vi "Answer Eval.vi"(5 "Answer Format":enum16{"Wfm", "Sim Param"}(ring), 6 "Error Deviation (%)":dbl=5.0 format="%#_13g", 7 "Exercise Number":T1, 8 "error in":errorcluster, 9 "Data In":variant, 11 "Exercise Folder Path":path) -> (0 "error out":errorcluster, 2 "Response Array":bool[](array[boolean]), 3 "path":path)   [LabVIEW 2014]
uses:
  Ctls/ExerciseNumeration.ctl
  Ctls/t1q1.ctl
  Ctls/RCSim Controls.ctl
  Ctls/t1q2.ctl
  <vilib>/express/express analysis/Spectral/Block/exnSpectralBlock spectral measurements peak poly.vi
  <vilib>/express/express analysis/Spectral/Block/exnSpectralBlock spectral measurements peak WFM.vi
  <vilib>/express/express analysis/Spectral/XNode/ExpressSpectralMeasurementsBlockNode.xnode
panel:
  out "Waveform In FFT":cluster{"f0":dbl, "df":dbl, "magnitude":dbl[]}(graph)
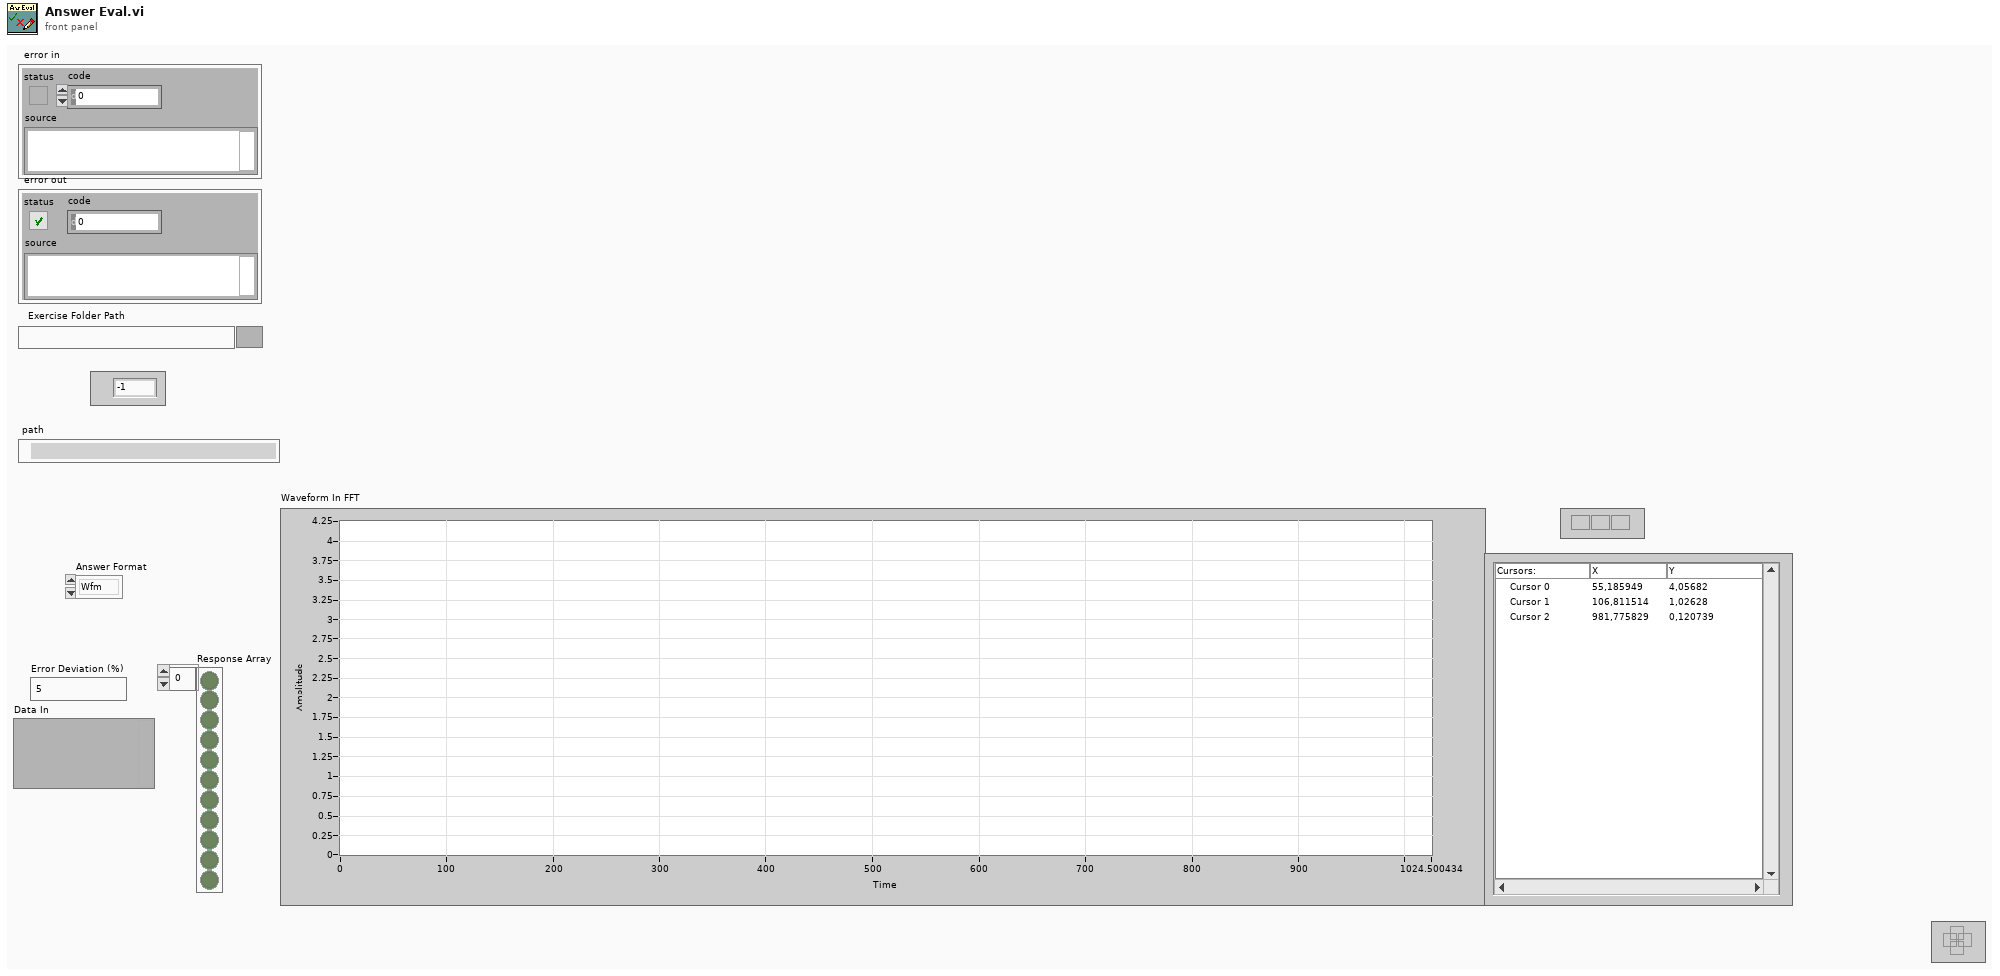
[diagram p1: front panel]
types:
  T1 = typedef "ExerciseNumeration.ctl" = enum16{"-1", "0", "1", "2", "3", "4", "5", "6", "7", "8", "9", "10"}
  T2 = cluster{"averaging mode":u16, "weighting mode":u16, "number of averages":u32}
  T3 = cluster{"dB On (F)":bool, "unwrap phase (F)":bool, "convert to degree (F)":bool}
  T4 = typedef "t1q1.ctl" = cluster{"Vsig (V)":dbl, "Fsig (Hz)":dbl, "Duty Cycle (%)":dbl, "R (Ohms)":dbl, "C (F)":dbl, "L (H)":dbl, "Circuit Type":enum16{"RL", "RC"}}
  T5 = enum16{"open", "replace", "create", "open or create", "replace or create", "replace or create with confirmation"}
  T6 = typedef "RCSim Controls.ctl" = cluster{"V":dbl, "C":dbl, "R":dbl, "L":dbl, "RC/RL":bool, "F":dbl, "DCycle":dbl}
  T7 = typedef "t1q2.ctl" = cluster{"Vsig (V)":dbl, "Fsig (Hz)":dbl, "R (Ohms)":dbl, "C (F)":dbl, "Duty Cycle (%)":dbl}
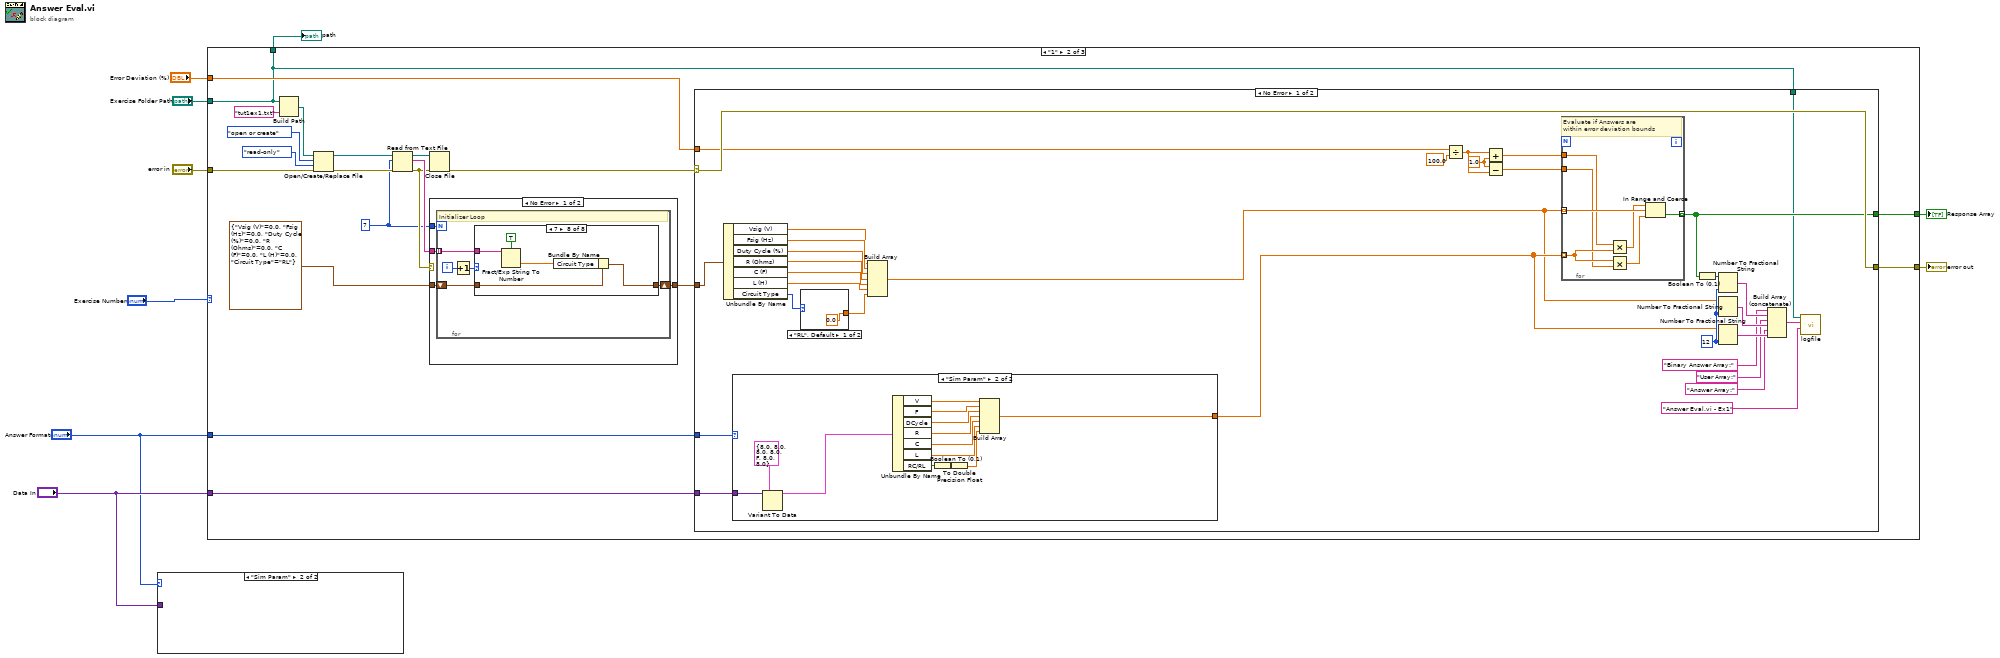
[diagram p0: block diagram]
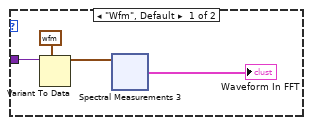
[diagram p2: hidden frame]
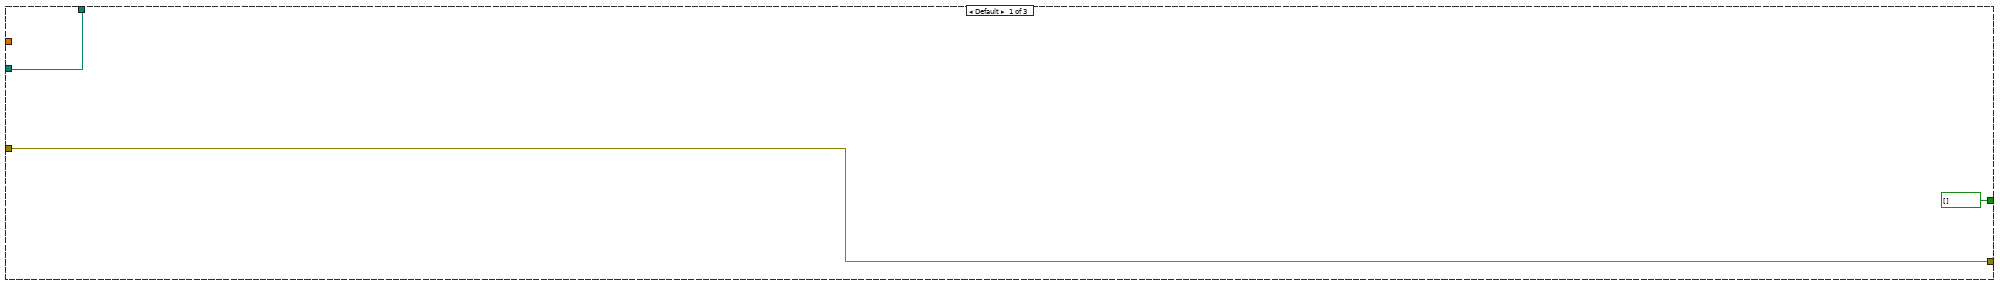
[diagram p3: hidden frame]
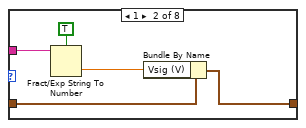
[diagram p5: hidden frame]
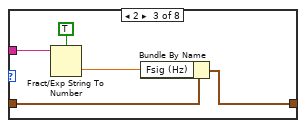
[diagram p6: hidden frame]
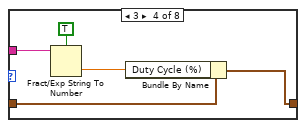
[diagram p7: hidden frame]
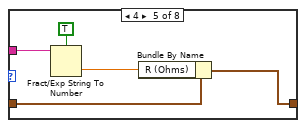
[diagram p8: hidden frame]
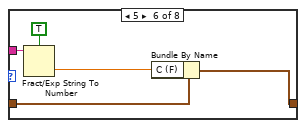
[diagram p9: hidden frame]
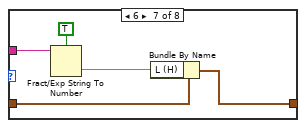
[diagram p10: hidden frame]
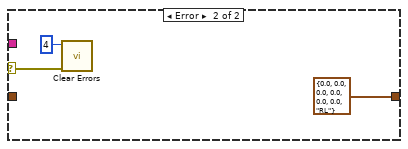
[diagram p11: hidden frame]
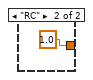
[diagram p12: hidden frame]
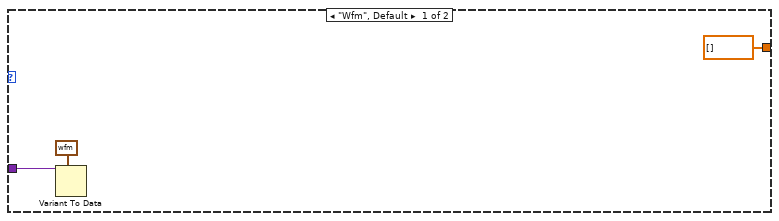
[diagram p13: hidden frame]
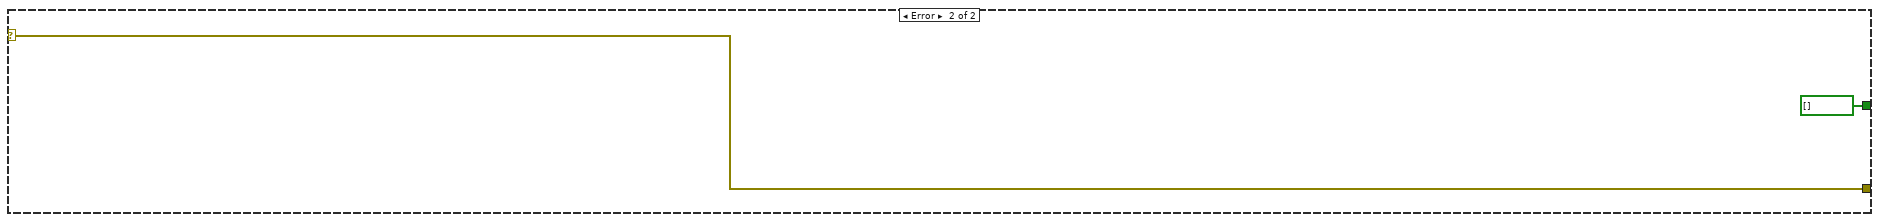
[diagram p14: hidden frame]
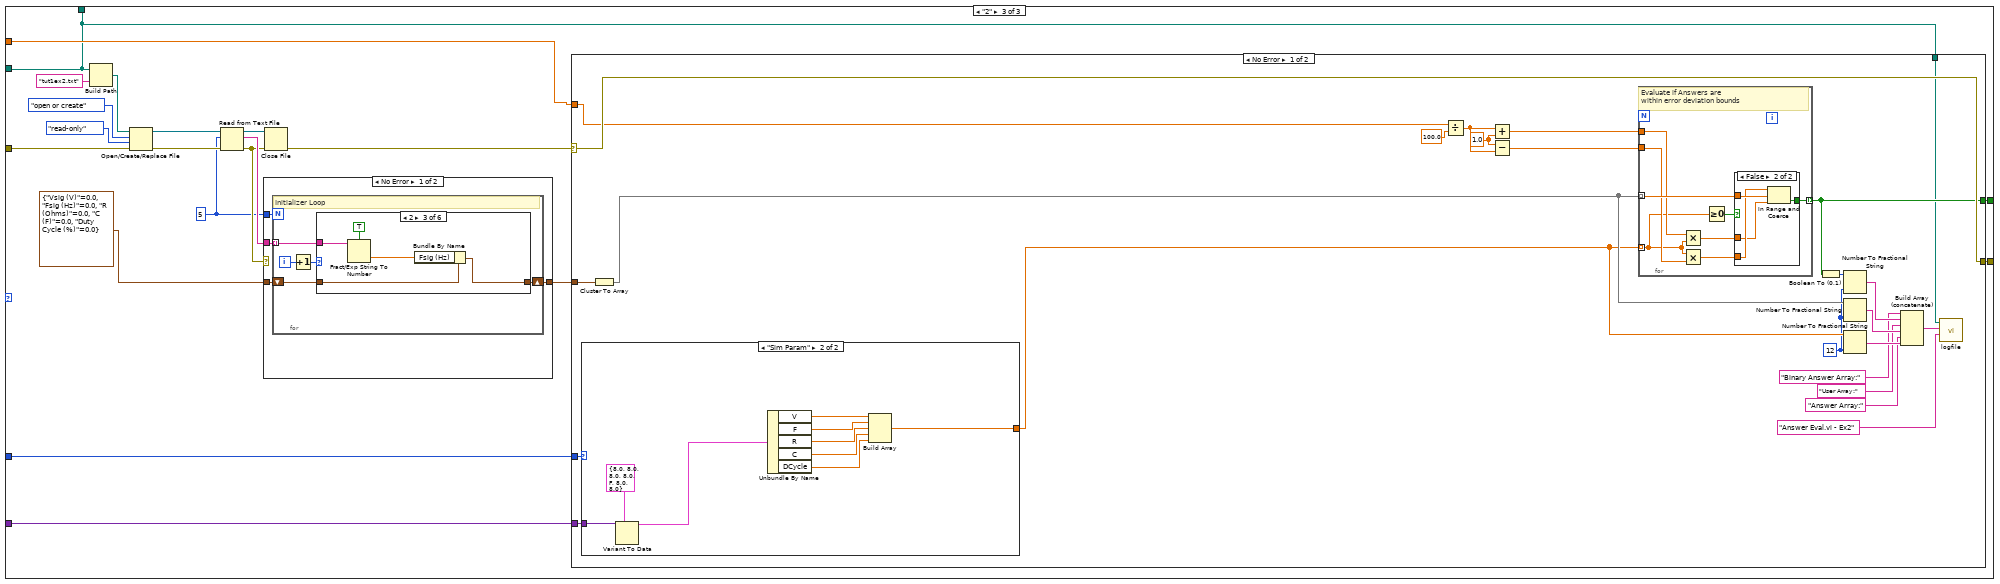
[diagram p15: hidden frame]
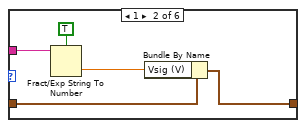
[diagram p17: hidden frame]
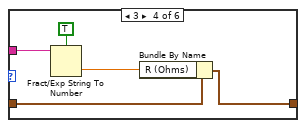
[diagram p18: hidden frame]
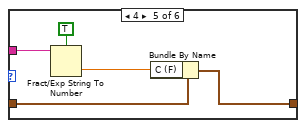
[diagram p19: hidden frame]
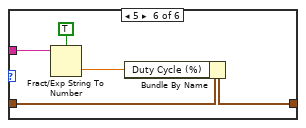
[diagram p20: hidden frame]
diagram:
  n1 = case shown="\"Sim Param\"" "Answer Format" {
    tunnel: "Data In" -> [w11 _]
    frame "Wfm", Default {
      n2 = Variant To Data(type=waveform(dbl) {"t0"=timestamp(0 s since 1904-01-01), "dt"=1.0, "Y"=[]} ("Waveform In"), Variant=w11) -> (data=w10:waveform(dbl))  [unwired: 1 in, 1 out]
      n3 = xnode "Spectral Measurements 3"("Signals"=w10) -> ("FFT - (Peak)"=→"Waveform In FFT":cluster{"f0":dbl, "df":dbl, "magnitude":dbl[]})  [unwired: 1 in, 2 out]
    }
    frame "Sim Param" {
    }
  }
  n4 = case shown="\"1\"" "Exercise Number" {
    tunnel: "Exercise Folder Path" -> [w25 w27 w154]
    tunnel: "error in" -> [w26 w44 w171]
    tunnel: [w26 w39 w166] -> w6
    tunnel: [w25 w27 w154] -> w7
    tunnel: "Error Deviation (%)" -> [_ w33 w160]
    tunnel: [bool[] [] w32 w159] -> w4
    tunnel: "Data In" -> [_ w31 w157]
    tunnel: "Answer Format" -> [_ w30 w156]
    frame Default {
    }
    frame "1" {
      w28 = 7
      n5 = Build Path(base path=w27, name or relative path="tut1ex1.txt") -> (appended path=w45:path)
      n6 = Open/Create/Replace File(file path (use dialog)=w45, error in=w44, operation (0:open)=T5."open or create", access (0:read/write)=enum16{"read/write", "read-only", "write-only"}."read-only") -> (refnum out=w41:refnum<file>, error out=w40:errorcluster)  [unwired: 2 in, 1 out]
      n7 = Read from Text File(file (use dialog)=w41, count=w28, error in=w40) -> (refnum out=w35:refnum<file>, text=w38:string[], error out=w36:errorcluster)  [unwired: 1 in, 1 out]
      n8 = case shown="No Error" w36 {
        selector: w36 -> [_ w94]
        tunnel: w38 -> [w50 _]
        tunnel: w28 -> [w49 _]
        tunnel: T4 {"Vsig (V)"=0.0, "Fsig (Hz)"=0.0, "Duty Cycle (%)"=0.0, "R (Ohms)"=0.0, "C (F)"=0.0, "L (H)"=0.0, "Circuit Type"=enum."RL"} ("T1E1") -> [w48 _]
        tunnel: [w47 T4 {"Vsig (V)"=0.0, "Fsig (Hz)"=0.0, "Duty Cycle (%)"=0.0, "R (Ohms)"=0.0, "C (F)"=0.0, "L (H)"=0.0, "Circuit Type"=enum."RL"} ("T1E1")] -> w37
        frame No Error {
          n9 = for {
            N: w49 -> [_]
            tunnel: w50 -> [w55] mode=indexing
            shift-right: [w51] -> w47
            shift-left: w48 -> [w52]
            i -> [w53]
            # "Initializer Loop"
            n10 = Increment(x=w53) -> (x+1=w54:i32)
            n11 = case shown="7" w54 {
              tunnel: w55 -> [_ w61 w66 w71 w76 w81 w86 w91]
              tunnel: w52 -> [w56 w59 w64 w69 w74 w79 w84 w89]
              tunnel: [w56 w57 w62 w67 w72 w77 w82 w87] -> w51
              frame 0, Default {
              }
              frame 1 {
                n12 = Fract/Exp String To Number(use system decimal point (T)=TRUE, string=w61) -> (number=w58:dbl)  [unwired: 2 in, 1 out]
                n13 = Bundle By Name(cluster=w59, "Vsig (V)"=w58) -> (w57:T4)
              }
              frame 2 {
                n14 = Fract/Exp String To Number(use system decimal point (T)=TRUE, string=w66) -> (number=w63:dbl)  [unwired: 2 in, 1 out]
                n15 = Bundle By Name(cluster=w64, "Fsig (Hz)"=w63) -> (w62:T4)
              }
              frame 3 {
                n16 = Fract/Exp String To Number(use system decimal point (T)=TRUE, string=w71) -> (number=w68:dbl)  [unwired: 2 in, 1 out]
                n17 = Bundle By Name(cluster=w69, "Duty Cycle (%)"=w68) -> (w67:T4)
              }
              frame 4 {
                n18 = Fract/Exp String To Number(use system decimal point (T)=TRUE, string=w76) -> (number=w73:dbl)  [unwired: 2 in, 1 out]
                n19 = Bundle By Name(cluster=w74, "R (Ohms)"=w73) -> (w72:T4)
              }
              frame 5 {
                n20 = Fract/Exp String To Number(use system decimal point (T)=TRUE, string=w81) -> (number=w78:dbl)  [unwired: 2 in, 1 out]
                n21 = Bundle By Name(cluster=w79, "C (F)"=w78) -> (w77:T4)
              }
              frame 6 {
                n22 = Fract/Exp String To Number(use system decimal point (T)=TRUE, string=w86) -> (number=w83:dbl)  [unwired: 2 in, 1 out]
                n23 = Bundle By Name(cluster=w84, "L (H)"=w83) -> (w82:T4)
              }
              frame 7 {
                n24 = Fract/Exp String To Number(use system decimal point (T)=TRUE, string=w91) -> (number=w88:dbl)  [unwired: 2 in, 1 out]
                n25 = Bundle By Name(cluster=w89, "Circuit Type"=w88) -> (w87:T4)
              }
            }
          }
        }
        frame Error {
          n26 = call <vilib>:"Clear Errors.vi"("error in (no error)"=w94, "specific error code to clear (0: all)"=4) -> ()  [unwired: 4 in, 2 out]
        }
      }
      n27 = Close File(refnum=w35, error in=w36) -> (error out=w34:errorcluster)  [unwired: 1 out]
      n28 = case shown="No Error" w34 {
        selector: w34 -> [w126 w153]
        tunnel: [w126 w153] -> w39
        tunnel: w37 -> [w109 _]
        tunnel: w33 -> [w122 _]
        tunnel: [w98 bool[] []] -> w32
        tunnel: w31 -> [w119 _]
        tunnel: w30 -> [w118 _]
        tunnel: w27 -> [w95 _]
        frame No Error {
          w107 = i16 12 ("precision (6)")
          w125 = 1.0 ("x")
          n29 = Unbundle By Name(w109) -> ("Vsig (V)"=w112:dbl, "Fsig (Hz)"=w113:dbl, "Duty Cycle (%)"=w117:dbl, "R (Ohms)"=w116:dbl, "C (F)"=w115:dbl, "L (H)"=w114:dbl, "Circuit Type"=w111:enum16{"RL", "RC"})
          n30 = case shown="\"Sim Param\"" w118 {
            tunnel: w119 -> [w130 w144]
            tunnel: [dbl[] [] w132] -> w97
            frame "Wfm", Default {
              n31 = Variant To Data(type=waveform(dbl) {"t0"=timestamp(0 s since 1904-01-01), "dt"=1.0, "Y"=[]} ("Waveform In"), Variant=w130) -> ()  [unwired: 1 in, 2 out]
            }
            frame "Sim Param" {
              n32 = Variant To Data(type=T6 {"V"=8.0, "C"=8.0, "R"=8.0, "L"=8.0, "RC/RL"=FALSE, "F"=8.0, "DCycle"=8.0} ("RC/RL Sim Param"), Variant=w144) -> (data=w142:T6)  [unwired: 1 in, 1 out]
              n33 = Unbundle By Name(w142) -> ("V"=w139:dbl, "F"=w138:dbl, "DCycle"=w137:dbl, "R"=w136:dbl, "C"=w135:dbl, "L"=w134:dbl, "RC/RL"=w141:bool)
              n34 = Boolean To (0,1)(Boolean=w141) -> (0, 1=w140:i16)
              n35 = To Double Precision Float(number=w140) -> (double precision float=w133:dbl)
              n36 = Build Array(w139, w138, w137, w136, w135, w134, w133) -> (w132:dbl[])
            }
          }
          n37 = case shown="\"RL\", Default" w111 {
            tunnel: [0.0 ("y") 1.0 ("y")] -> w110
            frame "RL", Default {
            }
            frame "RC" {
            }
          }
          n38 = Build Array(w112, w113, w117, w116, w115, w114, w110) -> (w96:dbl[])
          n39 = Divide(x=w122, y=100.0) -> (x/y=w123:dbl)
          n40 = Add(x=w123, y=w125) -> (x+y=w121:dbl)
          n41 = Subtract(x=w125, y=w123) -> (x-y=w120:dbl)
          n42 = for {
            tunnel: w97 -> [w150] mode=indexing
            tunnel: w96 -> [w151] mode=indexing
            tunnel: w121 -> [w149]
            tunnel: w120 -> [w148]
            tunnel: [w145] -> w98 mode=indexing
            # "Evaluate if Answers are\nwithin error deviation bounds"
            n43 = Multiply(x=w149, y=w150) -> (x*y=w147:dbl)
            n44 = Multiply(x=w150, y=w148) -> (x*y=w146:dbl)
            n45 = In Range and Coerce(upper limit=w147, x=w151, lower limit=w146) -> (In Range?=w145:bool)  [unwired: 1 out]
          }
          n46 = Boolean To (0,1)(Boolean=w98) -> (0, 1=w108:i16[])
          n47 = Number To Fractional String(number=w108, precision (6)=w107) -> (F-format string=w106:string[])  [unwired: 2 in]
          n48 = Number To Fractional String(number=w96, precision (6)=w107) -> (F-format string=w105:string[])  [unwired: 2 in]
          n49 = Number To Fractional String(number=w97, precision (6)=w107) -> (F-format string=w104:string[])  [unwired: 2 in]
          n50 = Build Array (concatenate)("Binary Answer Array:", w106, "User Array:", w105, "Answer Array:", w104) -> (w100:string[])
          n51 = call "logfile.vi"("Locale"="Answer Eval.vi - Ex1", "Text In"=w100, "Path In"=w95) -> ()  [unwired: 7 in, 2 out]
        }
        frame Error {
        }
      }
    }
    frame "2" {
      w155 = 5
      n52 = Build Path(base path=w154, name or relative path="tut1ex2.txt") -> (appended path=w172:path)
      n53 = Open/Create/Replace File(file path (use dialog)=w172, error in=w171, operation (0:open)=T5."open or create", access (0:read/write)=enum16{"read/write", "read-only", "write-only"}."read-only") -> (refnum out=w168:refnum<file>, error out=w167:errorcluster)  [unwired: 2 in, 1 out]
      n54 = Read from Text File(file (use dialog)=w168, count=w155, error in=w167) -> (refnum out=w162:refnum<file>, text=w165:string[], error out=w163:errorcluster)  [unwired: 1 in, 1 out]
      n55 = case shown="No Error" w163 {
        selector: w163 -> [_ w211]
        tunnel: w165 -> [w177 _]
        tunnel: w155 -> [w176 _]
        tunnel: [w174 T7 {"Vsig (V)"=0.0, "Fsig (Hz)"=0.0, "R (Ohms)"=0.0, "C (F)"=0.0, "Duty Cycle (%)"=0.0} ("T1E2")] -> w164
        tunnel: T7 {"Vsig (V)"=0.0, "Fsig (Hz)"=0.0, "R (Ohms)"=0.0, "C (F)"=0.0, "Duty Cycle (%)"=0.0} ("T1E2") -> [w175 _]
        frame No Error {
          n56 = for {
            N: w176 -> [_]
            tunnel: w177 -> [w182] mode=indexing
            shift-right: [w178] -> w174
            shift-left: w175 -> [w179]
            i -> [w180]
            # "Initializer Loop"
            n57 = Increment(x=w180) -> (x+1=w181:i32)
            n58 = case shown="2" w181 {
              tunnel: w182 -> [_ w188 w193 w198 w203 w208]
              tunnel: w179 -> [w183 w186 w191 w196 w201 w206]
              tunnel: [w183 w184 w189 w194 w199 w204] -> w178
              frame 0, Default {
              }
              frame 1 {
                n59 = Fract/Exp String To Number(use system decimal point (T)=TRUE, string=w188) -> (number=w185:dbl)  [unwired: 2 in, 1 out]
                n60 = Bundle By Name(cluster=w186, "Vsig (V)"=w185) -> (w184:T7)
              }
              frame 2 {
                n61 = Fract/Exp String To Number(use system decimal point (T)=TRUE, string=w193) -> (number=w190:dbl)  [unwired: 2 in, 1 out]
                n62 = Bundle By Name(cluster=w191, "Fsig (Hz)"=w190) -> (w189:T7)
              }
              frame 3 {
                n63 = Fract/Exp String To Number(use system decimal point (T)=TRUE, string=w198) -> (number=w195:dbl)  [unwired: 2 in, 1 out]
                n64 = Bundle By Name(cluster=w196, "R (Ohms)"=w195) -> (w194:T7)
              }
              frame 4 {
                n65 = Fract/Exp String To Number(use system decimal point (T)=TRUE, string=w203) -> (number=w200:dbl)  [unwired: 2 in, 1 out]
                n66 = Bundle By Name(cluster=w201, "C (F)"=w200) -> (w199:T7)
              }
              frame 5 {
                n67 = Fract/Exp String To Number(use system decimal point (T)=TRUE, string=w208) -> (number=w205:dbl)  [unwired: 2 in, 1 out]
                n68 = Bundle By Name(cluster=w206, "Duty Cycle (%)"=w205) -> (w204:T7)
              }
            }
          }
        }
        frame Error {
          n69 = call <vilib>:"Clear Errors.vi"("error in (no error)"=w211, "specific error code to clear (0: all)"=4) -> ()  [unwired: 4 in, 2 out]
        }
      }
      n70 = Close File(refnum=w162, error in=w163) -> (error out=w161:errorcluster)  [unwired: 1 out]
      n71 = case shown="No Error" w161 {
        selector: w161 -> [w235 w265]
        tunnel: [w235 w265] -> w166
        tunnel: w164 -> [w234 _]
        tunnel: w160 -> [w230 _]
        tunnel: [w223 bool[] []] -> w159
        tunnel: w157 -> [w227 _]
        tunnel: w156 -> [w226 _]
        tunnel: w154 -> [w212 _]
        frame No Error {
          w221 = i16 12 ("precision (6)")
          w233 = 1.0 ("x")
          n72 = case shown="\"Sim Param\"" w226 {
            tunnel: w227 -> [w237 w247]
            tunnel: [dbl[] [] w239] -> w224
            frame "Wfm", Default {
              n73 = Variant To Data(type=waveform(dbl) {"t0"=timestamp(0 s since 1904-01-01), "dt"=1.0, "Y"=[]} ("Waveform In"), Variant=w237) -> ()  [unwired: 1 in, 2 out]
            }
            frame "Sim Param" {
              n74 = Variant To Data(type=T6 {"V"=8.0, "C"=8.0, "R"=8.0, "L"=8.0, "RC/RL"=FALSE, "F"=8.0, "DCycle"=8.0} ("RC/RL Sim Param"), Variant=w247) -> (data=w245:T6)  [unwired: 1 in, 1 out]
              n75 = Unbundle By Name(w245) -> ("V"=w244:dbl, "F"=w243:dbl, "R"=w242:dbl, "C"=w241:dbl, "DCycle"=w240:dbl)
              n76 = Build Array(w244, w243, w242, w241, w240) -> (w239:dbl[])
            }
          }
          n77 = Cluster To Array(cluster=w234) -> (array=w225:dbl[])
          n78 = Divide(x=w230, y=100.0) -> (x/y=w231:dbl)
          n79 = Add(x=w231, y=w233) -> (x+y=w229:dbl)
          n80 = Subtract(x=w233, y=w231) -> (x-y=w228:dbl)
          n81 = for {
            tunnel: w225 -> [w255] mode=indexing
            tunnel: w229 -> [w254]
            tunnel: w228 -> [w253]
            tunnel: [w250] -> w223 mode=indexing
            tunnel: w224 -> [w248] mode=indexing
            # "Evaluate if Answers are\nwithin error deviation bounds"
            n82 = Multiply(x=w254, y=w248) -> (x*y=w252:dbl)
            n83 = Multiply(x=w248, y=w253) -> (x*y=w251:dbl)
            n84 = Greater Or Equal To 0?(x=w248) -> (x >= 0?=w249:bool)
            n85 = case shown="False" w249 {
              tunnel: w255 -> [w259 w263]
              tunnel: w252 -> [w258 w260]
              tunnel: w251 -> [w257 w261]
              tunnel: [w256 w262] -> w250
              frame True {
                n86 = In Range and Coerce(upper limit=w258, x=w259, lower limit=w257) -> (In Range?=w256:bool)  [unwired: 1 out]
              }
              frame False {
                n87 = In Range and Coerce(upper limit=w261, x=w263, lower limit=w260) -> (In Range?=w262:bool)  [unwired: 1 out]
              }
            }
          }
          n88 = Boolean To (0,1)(Boolean=w223) -> (0, 1=w222:i16[])
          n89 = Number To Fractional String(number=w222, precision (6)=w221) -> (F-format string=w220:string[])  [unwired: 2 in]
          n90 = Number To Fractional String(number=w225, precision (6)=w221) -> (F-format string=w219:string[])  [unwired: 2 in]
          n91 = Number To Fractional String(number=w224, precision (6)=w221) -> (F-format string=w218:string[])  [unwired: 2 in]
          n92 = Build Array (concatenate)("Binary Answer Array:", w220, "User Array:", w219, "Answer Array:", w218) -> (w214:string[])
          n93 = call "logfile.vi"("Locale"="Answer Eval.vi - Ex2", "Text In"=w214, "Path In"=w212) -> ()  [unwired: 7 in, 2 out]
        }
        frame Error {
        }
      }
    }
  }
  "error out" <- w6
  "path" <- w7
  "Response Array" <- w4
